vi "Create_Graph_v1.0.vi"() -> ()   [LabVIEW 2018]
uses:
  <vilib>/Native 3D Graph/xcontrol/3DPC_SurfacePlot.xctl
panel:
  out "3D Graph":refnum<class "Base Datatype.lvclass">[](xcontrol)
  out "element 2":dbl format="%#.8g"
  out "element 3":dbl
  out "element":dbl
  in  "Выбор файла":path
  in  "Open":bool
  out "Загруженные данные:":string[][](table)=[["3", "FS10035937", "SP01E", "BB15", "MP56270101", "", "", "R", "", "", "", "", "", ""], ["4", "FS10035937", "SP01E", "BB16", "MP56270101", "", "", "R", "", "", "", "", "", ""], ["5", "", "SP02E", "1200", "MP56270101", "", "", "L", "", "", "", "", "", ""], ["6", "", "SP02E", "122", "MP56270101", "", "", "L", "", "", "", "", "", ""], ["7", "", "SP02E", "1220", "MP56270101", "", "", "L", "", "", "", "", "", ""]]
  in  "Array":string[][](array[string])
  in  "Загрузка Excel приложения":refnum<k7>
  in  "Excel._Worksheet 2":refnum<k7>
  # "1. Запустите проект. \n2. Нажмите на кнопку \"папка\". Выберите необходимый файл с данными.\n3. Нажмите на кнопку \"Загрузить\". Дождитесь обновления и отображения файлов в таблице.\n4. Вращайте и исследуйте 3D график."
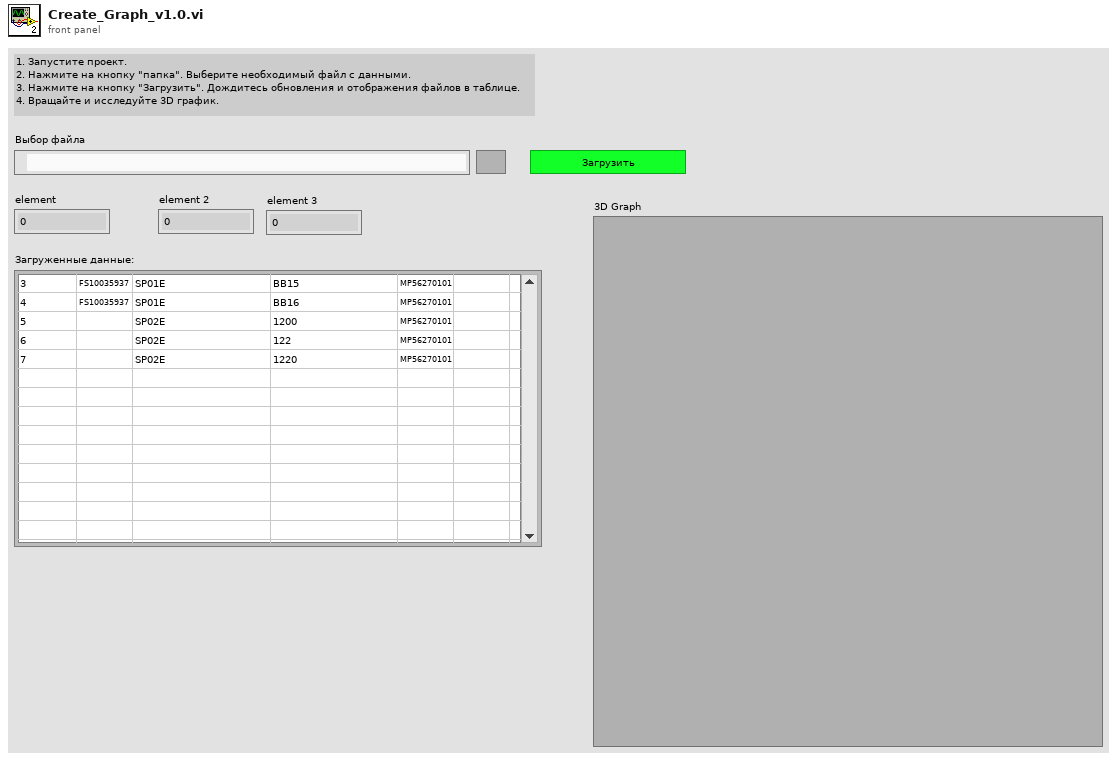
[diagram p1: front panel]
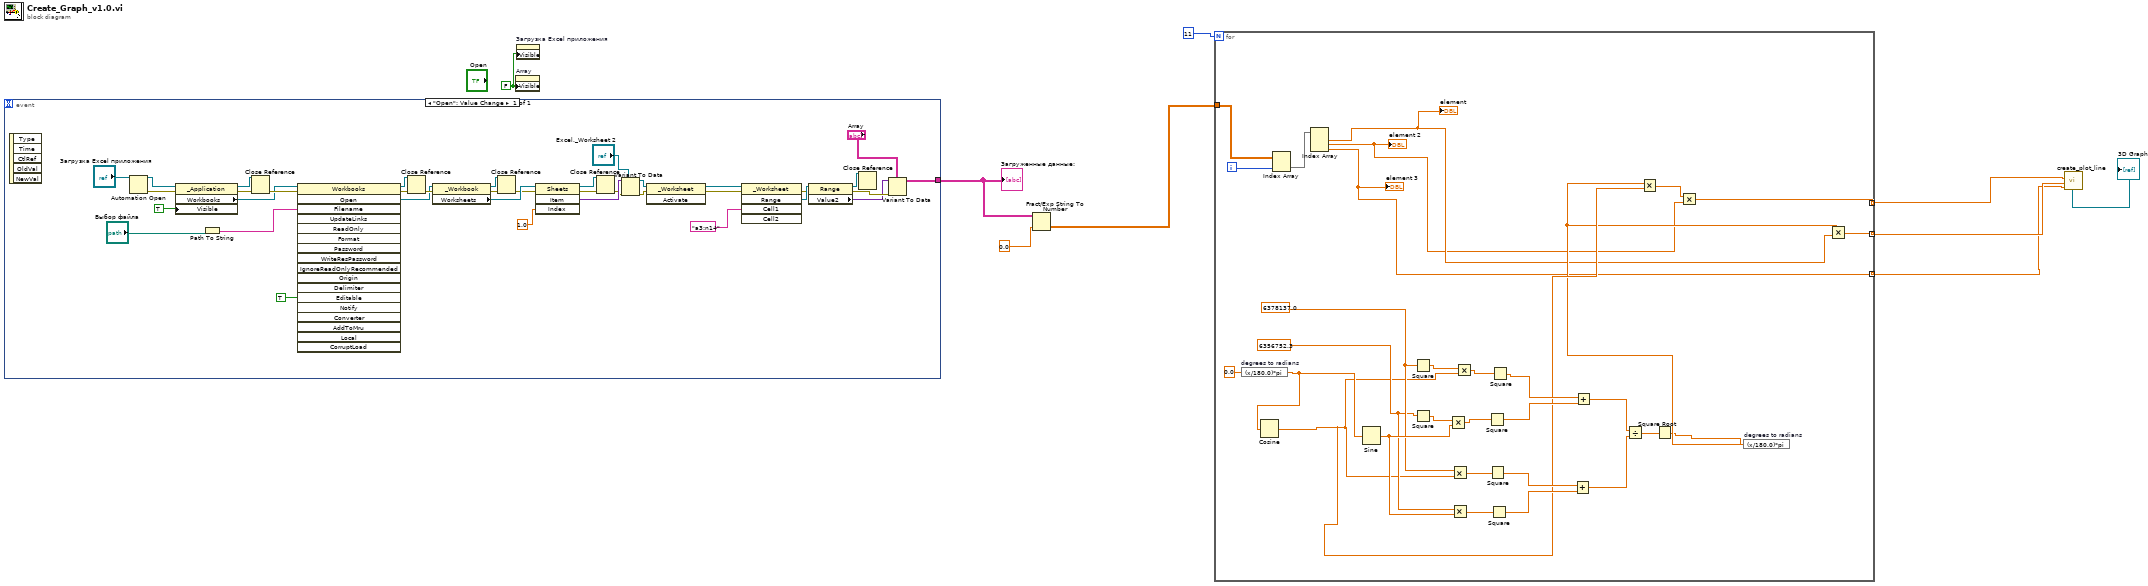
[diagram p0: block diagram]
diagram:
  w9 = FALSE ("Visible")
  n1 = event shown="[0] \"Open\": Value Change" {
    selector: _ -> [_]
    dyn-events: _ -> [_]
    timeout: _ -> [_]
    tunnel: [w13] -> w8
    event "Open": Value Change {
      n2 = event-data() -> ()  [unwired: 1 in, 5 out]
      n3 = Automation Open(Automation Refnum="Загрузка Excel приложения") -> (Automation Refnum=w46:refnum<k7>, error out=w33:errorcluster)  [unwired: 3 in]
      n4 = property class="_Application"(reference=w46, error in=w33, "Visible"=TRUE) -> (reference out=w31:refnum<k7>, error out=w26:errorcluster, "Workbooks"=w16:refnum<k7>)
      n5 = Path To String(path="Выбор файла") -> (string=w14:string)
      n6 = Close Reference(reference=w31, error in (no error)=w26) -> (error out=w25:errorcluster)
      n7 = invoke class="Workbooks" method="Open"(reference=w16, error in=w25, "Filename"=w14, "Editable"=TRUE) -> (reference out=w30:refnum<k7>, error out=w24:errorcluster, "Open"=w15:refnum<k7>)  [unwired: 14 in, 15 out]
      n8 = Close Reference(reference=w30, error in (no error)=w24) -> (error out=w23:errorcluster)
      n9 = property class="_Workbook"(reference=w15, error in=w23) -> (reference out=w29:refnum<k7>, error out=w22:errorcluster, "Worksheets"=w41:refnum<k7>)
      n10 = Close Reference(reference=w29, error in (no error)=w22) -> (error out=w21:errorcluster)
      n11 = invoke class="Sheets" method="Item"(reference=w41, error in=w21, "Index"=1.0) -> (reference out=w28:refnum<k7>, error out=w20:errorcluster, "Item"=w42:variant)  [unwired: 1 in, 1 out]
      n12 = Close Reference(reference=w28, error in (no error)=w20) -> (error out=w19:errorcluster)
      n13 = Variant To Data(error in=w19, type="Excel._Worksheet 2", Variant=w42) -> (data=w44:refnum<k7>, error out=w32:errorcluster)
      n14 = invoke class="_Worksheet" method="Activate"(reference=w44, error in=w32) -> (reference out=w35:refnum<k7>, error out=w18:errorcluster)  [unwired: 1 in, 1 out]
      n15 = invoke class="_Worksheet" method="Range"(reference=w35, error in=w18, "Cell1"="a3:n14") -> (error out=w17:errorcluster, "Range"=w37:refnum<k7>)  [unwired: 2 in, 3 out]
      n16 = property class="Range"(reference=w37, error in=w17) -> (reference out=w27:refnum<k7>, error out=w39:errorcluster, "Value2"=w38:variant)
      n17 = Close Reference(reference=w27) -> ()  [unwired: 1 in, 1 out]
      n18 = Variant To Data(error in=w39, type="Array", Variant=w38) -> (data=w13:string[][])  [unwired: 1 out]
    }
  }
  "Загруженные данные:" <- w8
  n19 = property on="Array" class="Arr (strict)"("Visible"=w9) -> ()  [unwired: 2 in, 2 out]
  n20 = property on="Загрузка Excel приложения" class="Ref (strict)"("Visible"=w9) -> ()  [unwired: 2 in, 2 out]
  n21 = Fract/Exp String To Number(string=w8, default (0 dbl)=0.0) -> (number=w1:dbl[][])  [unwired: 2 in, 1 out]
  n22 = for {
    N: 11 -> [_]
    tunnel: w1 -> [w74]
    tunnel: [w53] -> w4 mode=indexing
    tunnel: [w52] -> w3 mode=indexing
    tunnel: [w48] -> w2 mode=indexing
    i -> [w76]
    w61 = 6378137.0
    w58 = 6356752.3
    n23 = expression code="(x/180.0)*pi" "degrees to radians"(0.0) -> (w63:dbl)
    n24 = Cosine(x=w63) -> (cos(x)=w56:dbl)
    n25 = Index Array(array=w74, index (row)=w76) -> (element=w75:dbl[])  [unwired: 1 in]
    n26 = Index Array(array=w75) -> (element #1=w50:dbl, element #2=w49:dbl, element #3=w48:dbl)  [unwired: 3 in]
    "element 2" <- w49
    "element 3" <- w48
    "element" <- w50
    n27 = Sine(x=w63) -> (sin(x)=w70:dbl)
    n28 = Square(x=w61) -> (x^2=w62:dbl)
    n29 = Square(x=w58) -> (x^2=w57:dbl)
    n30 = Multiply(x=w57, y=w70) -> (x*y=w73:dbl)
    n31 = Multiply(x=w61, y=w56) -> (x*y=w71:dbl)
    n32 = Multiply(x=w58, y=w70) -> (x*y=w69:dbl)
    n33 = Multiply(x=w62, y=w56) -> (x*y=w60:dbl)
    n34 = Square(x=w73) -> (x^2=w72:dbl)
    n35 = Square(x=w71) -> (x^2=w68:dbl)
    n36 = Square(x=w69) -> (x^2=w67:dbl)
    n37 = Square(x=w60) -> (x^2=w59:dbl)
    n38 = Add(x=w68, y=w67) -> (x+y=w65:dbl)
    n39 = Add(x=w59, y=w72) -> (x+y=w66:dbl)
    n40 = Divide(x=w66, y=w65) -> (x/y=w64:dbl)
    n41 = Square Root(x=w64) -> (sqrt(x)=w47:dbl)
    n42 = expression code="(x/180.0)*pi" "degrees to radians"(w47) -> (w54:dbl)
    n43 = Multiply(x=w54, y=w56) -> (x*y=w55:dbl)
    n44 = Multiply(x=w55, y=w49) -> (x*y=w53:dbl)
    n45 = Multiply(x=w54, y=w50) -> (x*y=w52:dbl)
  }
  n46 = call <vilib>:"create_plot_line.vi"("z vector"=w2, "y vector"=w3, "x vector"=w4) -> ("plots out"=→"3D Graph":refnum<class "Base Datatype.lvclass">[])  [unwired: 2 in, 6 out]
